vi "PollStatusEnable.vi"(8 "error in (no error)":errorcluster, 10 "PollEnable":bool, 11 "TopLevel in":refnum<class "TopLevel.lvclass">) -> (0 "error out":errorcluster, 3 "TopLevel out":refnum<class "TopLevel.lvclass">)   [LabVIEW 2022 SP3, in "TopLevel.lvclass"]
uses:
  TopLevel.lvclass
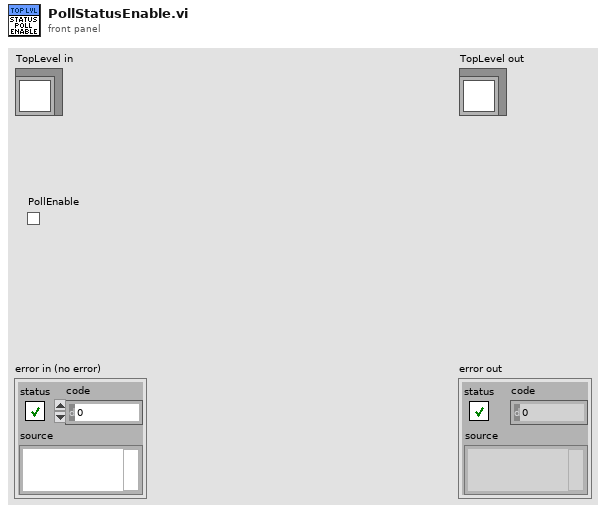
[diagram p1: front panel]
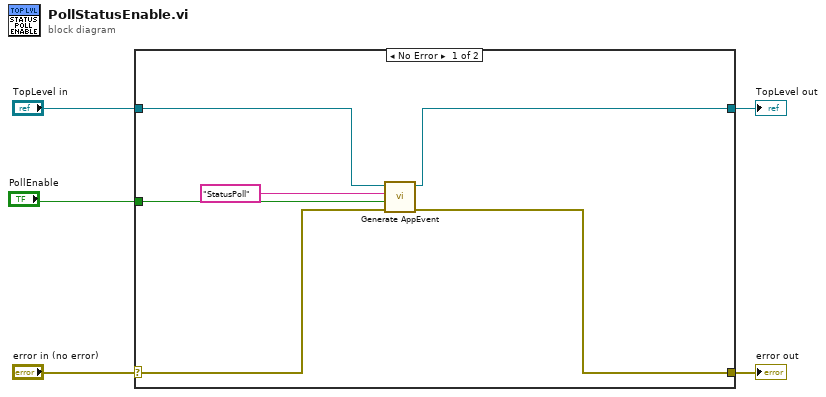
[diagram p0: block diagram]
diagram:
  n1 = case shown="No Error" "error in (no error)" {
    selector: "error in (no error)" -> [w9 w13]
    tunnel: [w8 w13] -> w4
    tunnel: [w11 w12] -> w2
    tunnel: "TopLevel in" -> [w10 w12]
    tunnel: "PollEnable" -> [w6 _]
    frame No Error {
      n2 = call-dynamic "Generate AppEvent.vi"("error in (no error)"=w9, "Data"=w6, "Command"="StatusPoll", "TopLevel in"=w10) -> ("error out"=w8:errorcluster, "TopLevel out"=w11:refnum<class "TopLevel.lvclass">)  [unwired: 6 in]
    }
    frame Error {
    }
  }
  "error out" <- w4
  "TopLevel out" <- w2
